vi "MathOptim-Power 2 Model.vi"(3 "output control":T1, 4 "data":variant, 5 "X":dbl[](array[numeric]), 6 "a":dbl[](array[numeric])) -> (0 "error out":errorcluster, 1 "f'(X,a)":dbl[][](array[numeric]), 2 "f(X,a)":dbl[](array[numeric]))   [LabVIEW 2020]
doc: "This template is the starting point for creating a model function to be passed to the Nonlinear Curve Fit.vi."
uses:
  <vilib>/gmath/NumericalOptimization/LM_output select.ctl
  <vilib>/Analysis/7linalg.llb/Solve Linear Equations (single right hand).vi
  <vilib>/Analysis/baseanly.llb/Solve Linear Equations By Cholesky.vi
  <vilib>/Analysis/baseanly.llb/Real Matrix to Compact Array.vi
  <vilib>/Analysis/baseanly.llb/Real Compact Tri-Matrix Linear Eqs.vi
  <vilib>/Analysis/7linalg.llb/Solve Linear Eqs (General).vi
  <vilib>/Analysis/7linalg.llb/Solve Linear Eqs (Gen, single right hand).vi
  <vilib>/Analysis/NI_AALPro.lvlib
  <vilib>/gmath/NI_Gmath.lvlib
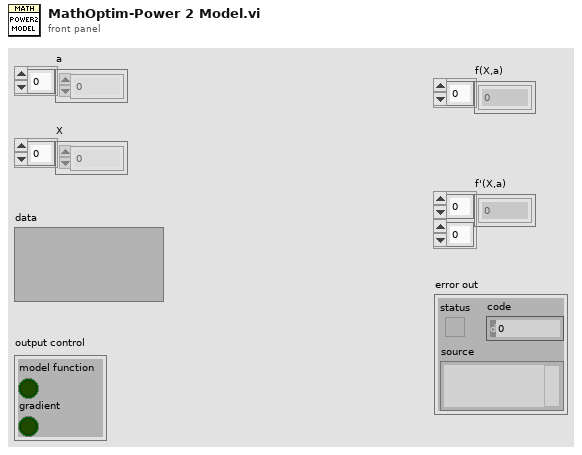
[diagram p1: front panel]
types:
  T1 = typedef "NI_Gmath.lvlib/LM_output select.ctl" = cluster{"model function":bool, "gradient":bool}
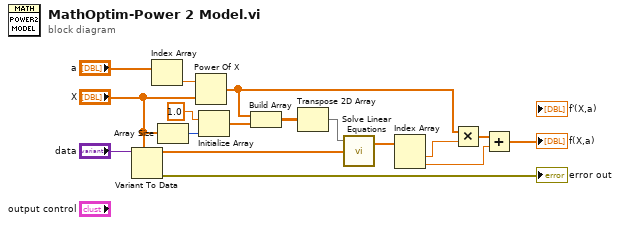
[diagram p0: block diagram]
diagram:
  n1 = Variant To Data(type="X", Variant="data") -> (data=w13:dbl[], error out=→"error out":errorcluster)  [unwired: 1 in]
  n2 = Index Array(array="a") -> (element=w14:dbl)  [unwired: 1 in]
  n3 = Array Size(array="X") -> (size(s)=w12:i32)
  n4 = Power Of X(1:"X", 2:w14) -> (0:w1:dbl[])
  n5 = Initialize Array(1.0, w12) -> (w10:dbl[])
  n6 = Build Array(w1, w10) -> (w9:dbl[][])
  n7 = Transpose 2D Array(2D array=w9) -> (transposed array=w2:dbl[][])
  n8 = call-poly <vilib>:"Solve Linear Equations.vi"("Known Vector"=w13, "Input Matrix"=w2) -> ("Solution Vector"=w8:dbl[])  [unwired: 1 in, 1 out]
  n9 = Index Array(array=w8) -> (element #1=w6:dbl, element #2=w4:dbl)  [unwired: 2 in]
  n10 = Multiply(x=w1, y=w6) -> (x*y=w5:dbl[])
  n11 = Add(x=w5, y=w4) -> (x+y=→"f(X,a)":dbl[])
